vi "Start TCP AI.vi"(8 "error in (no error)":errorcluster, 9 "Scans per Sample":i32=1 min=1, 10 "channel indices":i32[](array[numeric]), 11 "Connection ID in":refnum<k5>) -> (0 "error out":errorcluster, 1 "channels":i32, 3 "Connection ID out":refnum<k5>)   [LabVIEW 2019]
doc: "Opens the data transmission from the data server using the selected channels and scans per sample. A command containing the channel and scan information is sent to the data server via TCP. Data transmission from the data server begins immediately and thus this VI needs to be followed by a VI that reads the transmitted data.\n\nInputs\n\nConnection ID in - TCP connection\n\nChannel indices - Array of channel numbers. The channels can be in any order and can even be duplicated. The channel numbers refer to the index of the channel as it is being acquired by the data server. The Server Stats control in the Logon TCP AI VI can be used to determine the indexes of the channels being monitored by the data server.\n\nScans per sample - The number of scans the data server should make per scan that is actually transmitted to the client. The actual data frequency can be determined by using the information in the Server Stats control.\n\nError in - \n\nOutputs\n\nConnection ID out - TCP connection (the same one that came in!).\n\nchannels - The number of channels that are being monitored. This information is required by the Read TCP AI VI so the size of the TCP data transmissions can be determined.\n\nError out - Will flag any errors that occured in the TCP communication.\n\nCreated by Monroe Weber-Shirk\nCornell University\nmw24@cornell.edu\nJanuary 2000"
uses:
  DataServer/command cluster.ctl
  DataServer/command.ctl
panel:
  in  "command interface":T1={"command"=enum."Idle", "start time (ms)"=0, "Channel Indices"=[], "Scans per Sample"=1} {"Scans per Sample" min=1}
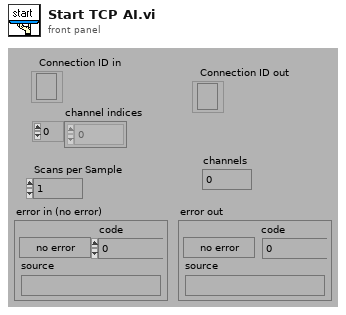
[diagram p1: front panel]
types:
  T1 = typedef "command cluster.ctl" = cluster{"command":T2, "start time (ms)":u32, "Channel Indices":i32[], "Scans per Sample":i32}
  T2 = typedef "command.ctl" = enum16{"Idle", "Send Data", "Send 1 Scan", "Logoff"}
  T3 = enum16{"Idle", "Send Data", "Send 1 Scan", "Logoff"}
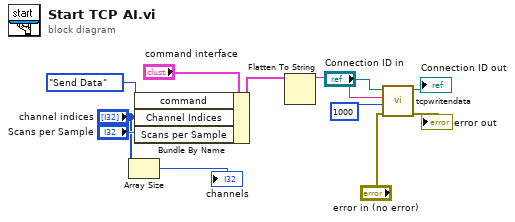
[diagram p0: block diagram]
diagram:
  n1 = Array Size(array="channel indices") -> (size(s)=→"channels":i32)
  n2 = Bundle By Name(cluster="command interface", "command"=T3."Send Data", "Channel Indices"="channel indices", "Scans per Sample"="Scans per Sample") -> (w7:T1)
  n3 = Flatten To String(anything=w7) -> (data string=w9:string)  [unwired: 3 in, 2 out]
  n4 = call "tcpwritendata.vi"("error in (no error)"="error in (no error)", "timeout ms (25000)"=1000, "data in"=w9, "refnum in"="Connection ID in") -> ("error out"=→"error out":errorcluster, "refnum out"=→"Connection ID out":refnum<k5>)  [unwired: 5 in, 1 out]
